vi "GetMessagesToRegister.vi"() -> (3 "subscribed messages":string[](array[string]))   [LabVIEW 2017, in "FileManager.lvlib"]
uses:
  <vilib>/addons/InsightCM/Devices/Shared/Common/FileManager/FileManager.lvlib
  <vilib>/addons/InsightCM/Devices/Shared/Common/ServerComm/ServerComm.lvlib
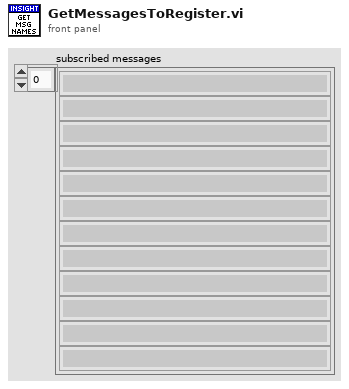
[diagram p1: front panel]
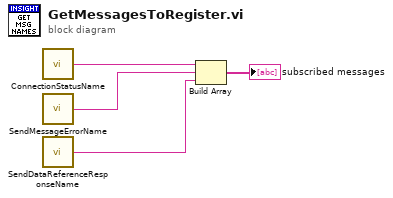
[diagram p0: block diagram]
diagram:
  n1 = call <vilib>:"ConnectionStatusName.vi"() -> ("message name"=w3:string)  [unwired: 5 in]
  n2 = call <vilib>:"SendMessageErrorName.vi"() -> ("message name"=w2:string)  [unwired: 5 in]
  n3 = call <vilib>:"SendDataReferenceResponseName.vi"() -> ("message name"=w1:string)  [unwired: 5 in]
  n4 = Build Array(w3, w2, w1) -> (→"subscribed messages":string[])
